vi "Fill.vi"(6 "Color":u32(colorbox), 8 "error in (no error)":errorcluster, 9 "point(x,y)":cluster{"x":i16, "y":i16}, 10 "Ref Color":u32(colorbox), 11 "Data in":T1={"Class"={"Ants"=refnum, "Layer"=refnum, "Templates"=refnum, "Icon"=refnum, "Glyph"=refnum, "Settings"=refnum, "Tools"=refnum}, "Ref"={"Add Layer"=refnum, "Remove Layer"=refnum, "Line Text"=[], "Body Text Spec"=refnum, "DNL_Font"=refnum, "glyph path str"=refnum, "templates path str"=refnum, "Arrow Up"=refnum, "Arrow Down"=refnum, "IE VI Ref"=refnum, "Glyphs tree"=refnum, "Templates tree"=refnum, "Layer Icon Text"=refnum, "Layer Template"=refnum, "Clipboard"=refnum, "BW icon in"=refnum, "Color icon in"=refnum, "Layer Clust"=refnum, "Body Text"=refnum, "DNL_Framework Templates"=refnum, "Search Templates"=refnum, "TextMarker"=refnum, "Tab Control"=refnum, "Search Glyphs"=refnum, "Line Color"=refnum, "DNL_Glyphs []"=refnum, "Fill Color"=refnum, "Tools"=refnum, "Glyphs tree"=refnum, "Icon"=refnum, "Preview"=refnum, "Ants"=refnum, "Terminals"=refnum, "menu reference"=refnum, "LayerNames"=[], "GlyphLoadAnimation"=refnum, "TemplateLoadAnimation"=refnum, "refreshGlyphs"=refnum, "refreshTemplates"=refnum}, "Support"={"AntsRect"={"left"=0, "top"=0, "right"=0, "bottom"=0}, "Mouse Move Coords"={"Horizontal"=0, "Vertical"=0}, "Mouse Down Coords"={"Horizontal"=0, "Vertical"=0}, "Temp Coord"={"Horizontal"=0, "Vertical"=0}, "Action"=enum."Default", "Edge Color"=4914962, "Fill Color"=16860, "Mouse Down?"=FALSE, "Draft Mode?"=FALSE, "Temp Icon"=bytes[3102], "CTRL Pressed"=FALSE, "Move Selection?"=FALSE, "AntsRect Orig"={"left"=0, "top"=0, "right"=0, "bottom"=0}, "Text"="", "TM Set?"=FALSE, "Mouse inside icon?"=FALSE, "Tool (old value)"=0, "Pencil Move Color"=0, "Swap Colors?"=FALSE, "Shift pressed?"=FALSE}}) -> (0 "error out":errorcluster, 3 "Data out":T1={"Class"={"Ants"=refnum, "Layer"=refnum, "Templates"=refnum, "Icon"=refnum, "Glyph"=refnum, "Settings"=refnum, "Tools"=refnum}, "Ref"={"Add Layer"=refnum, "Remove Layer"=refnum, "Line Text"=[], "Body Text Spec"=refnum, "DNL_Font"=refnum, "glyph path str"=refnum, "templates path str"=refnum, "Arrow Up"=refnum, "Arrow Down"=refnum, "IE VI Ref"=refnum, "Glyphs tree"=refnum, "Templates tree"=refnum, "Layer Icon Text"=refnum, "Layer Template"=refnum, "Clipboard"=refnum, "BW icon in"=refnum, "Color icon in"=refnum, "Layer Clust"=refnum, "Body Text"=refnum, "DNL_Framework Templates"=refnum, "Search Templates"=refnum, "TextMarker"=refnum, "Tab Control"=refnum, "Search Glyphs"=refnum, "Line Color"=refnum, "DNL_Glyphs []"=refnum, "Fill Color"=refnum, "Tools"=refnum, "Glyphs tree"=refnum, "Icon"=refnum, "Preview"=refnum, "Ants"=refnum, "Terminals"=refnum, "menu reference"=refnum, "LayerNames"=[], "GlyphLoadAnimation"=refnum, "TemplateLoadAnimation"=refnum, "refreshGlyphs"=refnum, "refreshTemplates"=refnum}, "Support"={"AntsRect"={"left"=0, "top"=0, "right"=0, "bottom"=0}, "Mouse Move Coords"={"Horizontal"=0, "Vertical"=0}, "Mouse Down Coords"={"Horizontal"=0, "Vertical"=0}, "Temp Coord"={"Horizontal"=0, "Vertical"=0}, "Action"=enum."Default", "Edge Color"=4914962, "Fill Color"=16860, "Mouse Down?"=FALSE, "Draft Mode?"=FALSE, "Temp Icon"=bytes[3102], "CTRL Pressed"=FALSE, "Move Selection?"=FALSE, "AntsRect Orig"={"left"=0, "top"=0, "right"=0, "bottom"=0}, "Text"="", "TM Set?"=FALSE, "Mouse inside icon?"=FALSE, "Tool (old value)"=0, "Pencil Move Color"=0, "Swap Colors?"=FALSE, "Shift pressed?"=FALSE}})   [LabVIEW 2021, in "Tools Paint.lvclass"]
uses:
  <resource>/plugins/NIIconEditor/Class/Tools/Tools Paint.lvclass
  <resource>/plugins/NIIconEditor/Controls/IE Data.ctl
  <resource>/plugins/NIIconEditor/Class/Ants/Ants.lvclass
  <resource>/plugins/NIIconEditor/Class/FakedArray/FakedArray.lvclass
  <vilib>/LabVIEW Icon API/lv_icon/Classes/Icon/Icon.lvclass
  <resource>/plugins/NIIconEditor/Class/Icon Library/Glyph.lvclass
  <resource>/plugins/NIIconEditor/Class/Settings/Settings.lvclass
  <resource>/plugins/NIIconEditor/Controls/IE Classes.ctl
  <resource>/plugins/NIIconEditor/Controls/References Cluster.ctl
  <resource>/plugins/NIIconEditor/Controls/SupportClass.ctl
  <vilib>/Utility/miscctls.llb/LVPoint32TypeDef.ctl
  <resource>/plugins/NIIconEditor/Controls/SupportClass_Action.ctl
  <vilib>/LabVIEW Icon API/lv_icon/Controls/IEColor.ctl
  <vilib>/LabVIEW Icon API/lv_icon/Controls/LayerType.ctl
  <vilib>/LabVIEW Icon API/lv_icon/Classes/Layer/Layer.lvclass
  <vilib>/LabVIEW Icon API/lv_icon/Classes/Icon Framework/Icon Framework.lvclass
  C:/projects/labview-icon-editor/source/vi.lib/LabVIEW Icon API/lv_icon/Classes/Layer/Layer.lvclass
  <vilib>/LabVIEW Icon API/lv_icon/lv_icon.lvlib
panel:
  in  "Fill":string="Fill"
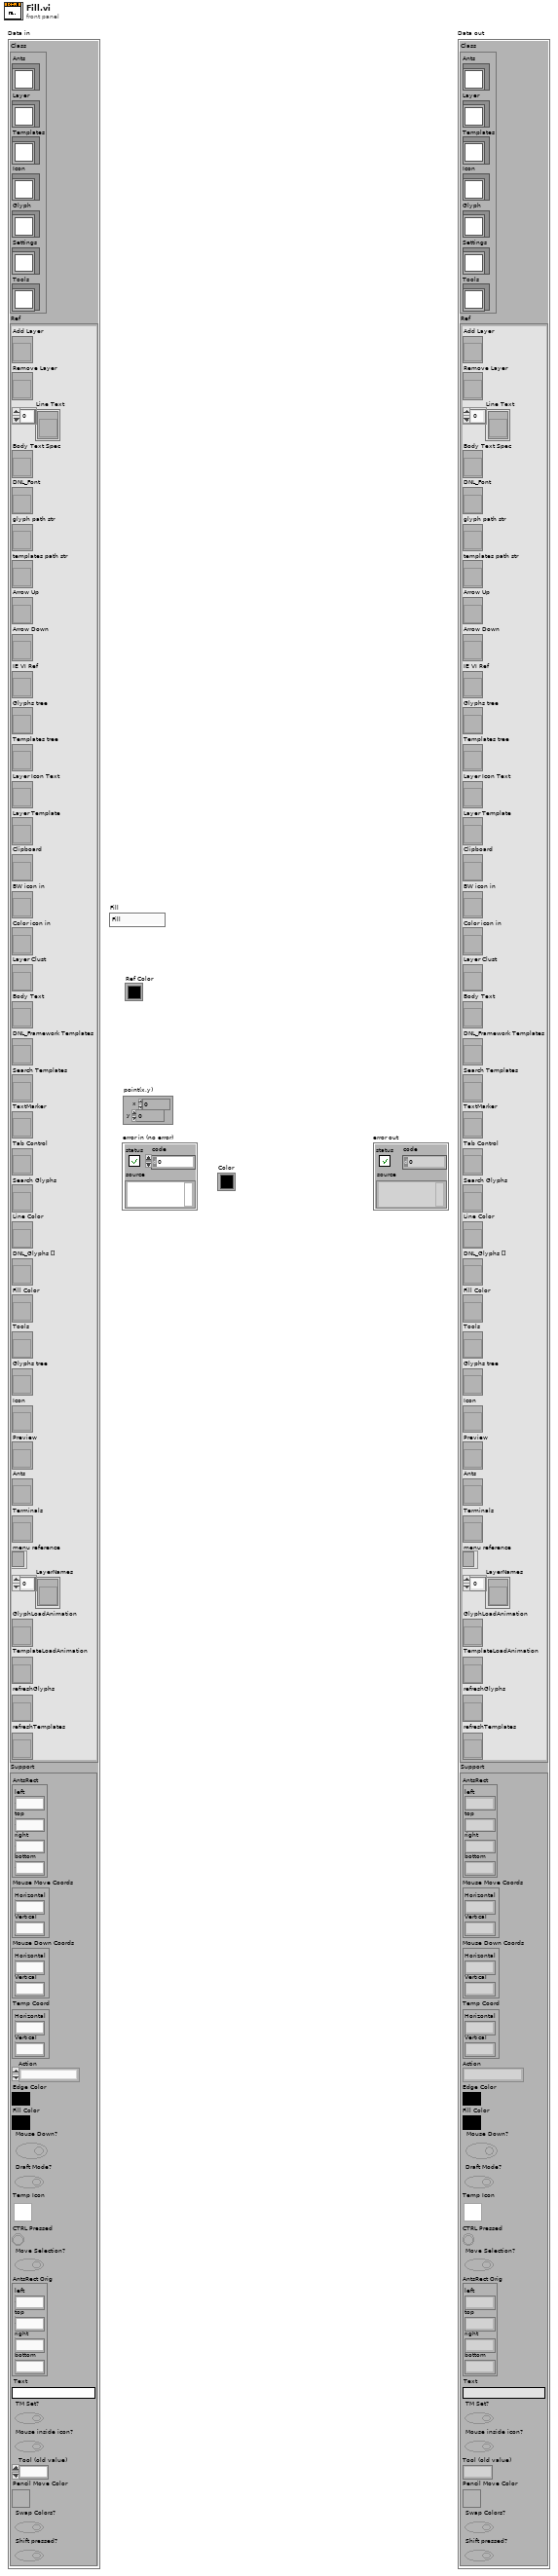
[diagram p1: front panel]
types:
  T1 = typedef "IE Data.ctl" = cluster{"Class":T2, "Ref":T3, "Support":T4}
  T2 = typedef "IE Classes.ctl" = cluster{"Ants":refnum<class "Ants.lvclass">, "Layer":refnum<class "FakedArray.lvclass">, "Templates":refnum<class "FakedArray.lvclass">, "Icon":refnum<class "Icon.lvclass">, "Glyph":refnum<class "Glyph.lvclass">, "Settings":refnum<class "Settings.lvclass">, "Tools":refnum<class "Tools Paint.lvclass">}
  T3 = typedef "References Cluster.ctl" = cluster{"Add Layer":refnum<vi>, "Remove Layer":refnum<vi>, "Line Text":refnum<vi>[], "Body Text Spec":refnum<vi>, "DNL_Font":refnum<vi>, "glyph path str":refnum<vi>, "templates path str":refnum<vi>, "Arrow Up":refnum<vi>, "Arrow Down":refnum<vi>, "IE VI Ref":refnum<vi>, "Glyphs tree":refnum<vi>, "Templates tree":refnum<vi>, "Layer Icon Text":refnum<vi>, "Layer Template":refnum<vi>, "Clipboard":refnum<vi>, "BW icon in":refnum<vi>, "Color icon in":refnum<vi>, "Layer Clust":refnum<vi>, "Body Text":refnum<vi>, "DNL_Framework Templates":refnum<vi>, "Search Templates":refnum<vi>, "TextMarker":refnum<vi>, "Tab Control":refnum<vi>, "Search Glyphs":refnum<vi>, "Line Color":refnum<vi>, "DNL_Glyphs []":refnum<vi>, "Fill Color":refnum<vi>, "Tools":refnum<vi>, "Glyphs tree":refnum<vi>, "Icon":refnum<vi>, "Preview":refnum<vi>, "Ants":refnum<vi>, "Terminals":refnum<vi>, "menu reference":refnum<k9>, "LayerNames":refnum<vi>[], "GlyphLoadAnimation":refnum<vi>, "TemplateLoadAnimation":refnum<vi>, "refreshGlyphs":refnum<vi>, "refreshTemplates":refnum<vi>}
  T4 = typedef "SupportClass.ctl" = cluster{"AntsRect":cluster{"left":i16, "top":i16, "right":i16, "bottom":i16}, "Mouse Move Coords":T5, "Mouse Down Coords":T5, "Temp Coord":T5, "Action":T6, "Edge Color":T7, "Fill Color":T7, "Mouse Down?":bool, "Draft Mode?":bool, "Temp Icon":picture, "CTRL Pressed":bool, "Move Selection?":bool, "AntsRect Orig":cluster{"left":i16, "top":i16, "right":i16, "bottom":i16}, "Text":string, "TM Set?":bool, "Mouse inside icon?":bool, "Tool (old value)":u32, "Pencil Move Color":u32, "Swap Colors?":bool, "Shift pressed?":bool}
  T5 = typedef "LVPoint32TypeDef.ctl" = cluster{"Horizontal":i32, "Vertical":i32}
  T6 = typedef "SupportClass_Action.ctl" = enum16{"Default", "Move Selection", "Glyph Library", "Tool"}
  T7 = typedef "IEColor.ctl" = u32
  T8 = typedef "LayerType.ctl" = enum16{"Graphic", "Text", "Tool", "Graphic Drop"}
  T9 = typedef "INI.ctl" = cluster{"Show Layer Tab?":bool, "Show Terminals?":bool, "Text":cluster{"Font":T10, "Alignment":T11, "Size":T12}, "3rd party Templates":cluster{"Store 3rd party Templates?":bool, "Folder Name":string}, "Merge user layers on commit":bool, "Body Text":T13, "Fill Color":T7, "Edge Color":T7, "Tab":u16, "Tool":T14, "Disable Layers?":bool}
  T10 = typedef "Font.ctl" = string
  T11 = typedef "Alignment.ctl" = u16
  T12 = typedef "Font Size.ctl" = u8
  T13 = typedef "BodyText.ctl" = cluster{"Line 1 text":string, "Line 2 text":string, "Line 3 text":string, "Line 4 text":string, "Line 1 color":u32, "Line 2 color":u32, "Line 3 color":u32, "Line 4 color":u32, "Body Text Spec":cluster{"Font":T10, "Alignment":T11, "Size":u8}, "Center text vertically":bool, "Capitalize Text":bool}
  T14 = typedef "Tools.ctl" = enum32{"Pencil", "Line", "Dropper", "Fill", "Rectangle", "Filled Rectangle", "Ellipse", "Filled Ellipse", "Eraser", "Text", "Select", "Move"}
  T15 = typedef "Layer.ctl" = cluster{"LayerIcon":picture, "LayerName":string, "Opacity":u8, "Visibility?":bool}
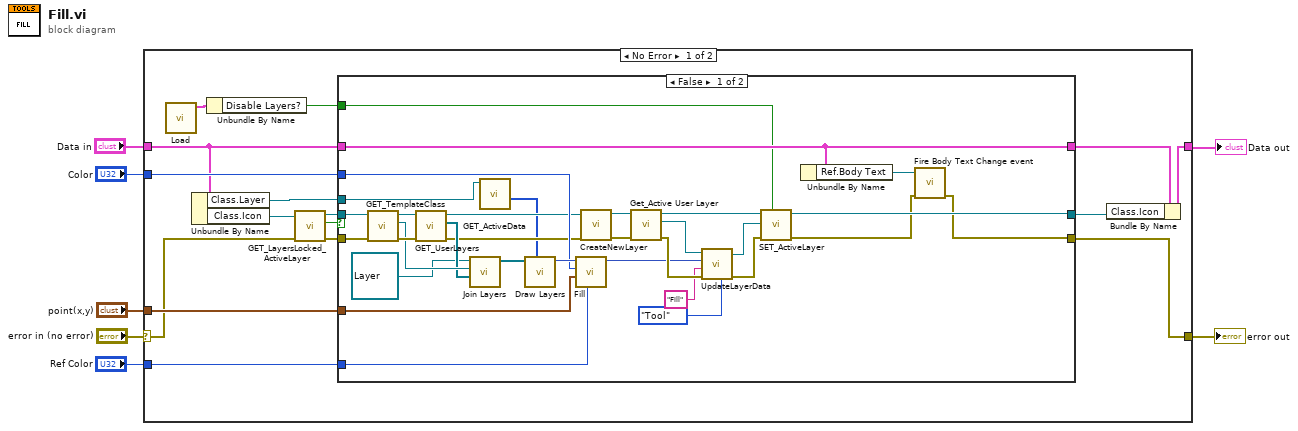
[diagram p0: block diagram]
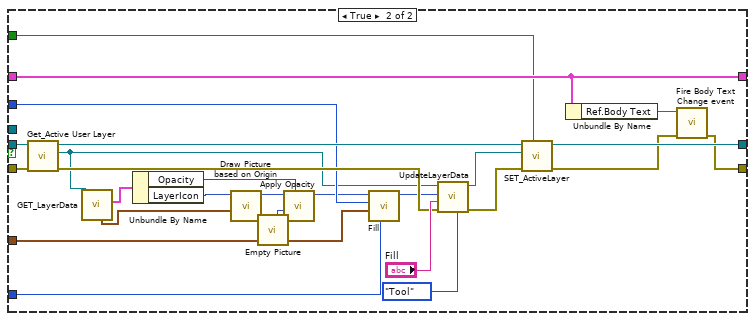
[diagram p2: hidden frame]
diagram:
  n1 = case shown="No Error" "error in (no error)" {
    selector: "error in (no error)" -> [w17 w83]
    tunnel: [w13 w83] -> w6
    tunnel: "point(x,y)" -> [w23 _]
    tunnel: "Color" -> [w19 _]
    tunnel: "Ref Color" -> [w18 _]
    tunnel: "Data in" -> [w15 w82]
    tunnel: [w12 w82] -> w1
    frame No Error {
      n2 = call <resource>:"Load.vi"() -> ("INI Data"=w9:T9)  [unwired: 2 in, 9 out]
      n3 = Unbundle By Name(w15) -> ("Class.Layer"=w10:refnum<class "FakedArray.lvclass">, "Class.Icon"=w16:refnum<class "Icon.lvclass">)
      n4 = Unbundle By Name(w9) -> ("Disable Layers?"=w8:bool)
      n5 = call-dynamic "GET_LayersLocked_ActiveLayer.vi"("error in (no error)"=w17, "Icon.lvclass in"=w16) -> ("error out"=w21:errorcluster, "Layers Locked?"=w20:bool, "Icon.lvclass out"=w22:refnum<class "Icon.lvclass">)  [unwired: 7 out]
      n6 = case shown="False" w20 {
        tunnel: w23 -> [w46 w72]
        tunnel: [w32 w79] -> w11
        tunnel: w22 -> [w54 w81]
        tunnel: w21 -> [w55 w80]
        tunnel: w19 -> [w47 w73]
        tunnel: w18 -> [w48 w71]
        tunnel: [w29 w58] -> w13
        tunnel: w15 -> [w28 w60]
        tunnel: [w28 w60] -> w14
        tunnel: w10 -> [w25 _]
        tunnel: w8 -> [w26 w56]
        frame False {
          n7 = call-dynamic "GET_TemplateClass.vi"("error in (no error)"=w55, "Icon.lvclass in"=w54) -> ("error out"=w53:errorcluster, "Icon Framework.lvclass"=w51:refnum<class "Icon Framework.lvclass">, "Icon.lvclass out"=w52:refnum<class "Icon.lvclass">)  [unwired: 7 out]
          n8 = call-dynamic "GET_UserLayers.vi"("error in (no error)"=w53, "Icon.lvclass in"=w52) -> ("error out"=w34:errorcluster, "All Layers"=w45:refnum<class "Layer.lvclass">[], "Icon.lvclass out"=w35:refnum<class "Icon.lvclass">)  [unwired: 7 out]
          n9 = call <vilib>:"Join Layers.vi"("User Layers"=w45, "Template"=w51, "Icon Text"=refnum<class "Layer.lvclass"> refnum) -> ("Layer out"=w50:refnum<class "Layer.lvclass">[])  [unwired: 3 in, 5 out]
          n10 = call-dynamic "GET_ActiveData.vi"("FakedArray in"=w25) -> ("Active Data []"=w24:i32[])  [unwired: 5 in, 5 out]
          n11 = call <vilib>:"Draw Layers.vi"("Active User Layer Data []"=w24, "Layers"=w50) -> ("Picture"=w49:picture)  [unwired: 3 in, 6 out]
          n12 = call <vilib>:"Fill.vi"("Ref Color"=w48, "Pic Mouse Down"=w46, "New Color"=w47, "Pic In"=w49) -> ("Pic Out"=w33:picture)  [unwired: 3 in, 4 out]
          n13 = call <vilib>:"CreateNewLayer.vi"("error in"=w34, "Icon.lvclass"=w35) -> ("error out"=w43:errorcluster, "Icon.lvclass out"=w44:refnum<class "Icon.lvclass">)  [unwired: 3 in, 5 out]
          n14 = call-dynamic "Get_Active User Layer.vi"("error in (no error)"=w43, "Icon in"=w44) -> ("error out"=w38:errorcluster, "Layer.lvclass"=w42:refnum<class "Layer.lvclass">, "Icon out"=w41:refnum<class "Icon.lvclass">)  [unwired: 7 out]
          n15 = call <vilib>:"UpdateLayerData.vi"("Type"=LayerType."Tool", "error in"=w38, "LayerName"="Fill" ("FileName"), "new picture"=w33, "Active Layer"=w42) -> ("error out"=w39:errorcluster, "Layer.lvclass out"=w40:refnum<class "Layer.lvclass">)  [unwired: 3 in, 2 out]
          n16 = call-dynamic "SET_ActiveLayer.vi"("Combine User Layers?"=w26, "error in (no error)"=w39, "Layer.lvclass"=w40, "Icon.lvclass in"=w41) -> ("error out"=w30:errorcluster, "Icon.lvclass out"=w32:refnum<class "Icon.lvclass">)  [unwired: 6 out]
          n17 = Unbundle By Name(w28) -> ("Ref.Body Text"=w27:refnum<vi>)
          n18 = call <resource>:"Fire Body Text Change event.vi"("error in"=w30, "Ref.Body Text"=w27) -> ("error out"=w29:errorcluster)  [unwired: 2 in, 7 out]
        }
        frame True {
          n19 = call-dynamic "Get_Active User Layer.vi"("error in (no error)"=w80, "Icon in"=w81) -> ("error out"=w75:errorcluster, "Layer.lvclass"=w66:refnum<class "Layer.lvclass">, "Icon out"=w78:refnum<class "Icon.lvclass">)  [unwired: 7 out]
          n20 = call-dynamic "GET_LayerData.vi"("Layer.lvclass in"=w66) -> ("Data"=w65:T15, "Origin"=w63:T5)  [unwired: 1 in, 8 out]
          n21 = Unbundle By Name(w65) -> ("Opacity"=w62:u8, "LayerIcon"=w64:picture)
          n22 = call <vilib>:"Draw Picture based on Origin.vi"("Origin"=w63, "LayerIcon in"=w64) -> ("LayerIcon out"=w67:picture)  [unwired: 1 in, 8 out]
          n23 = call "Empty Picture"() -> ("empty picture"=w68:picture)
          n24 = call <vilib>:"Apply Opacity.vi"("% (100)"=w62, "Bottom"=w68, "Top"=w67) -> ("new picture"=w61:picture)  [unwired: 8 out]
          n25 = call <vilib>:"Fill.vi"("Ref Color"=w71, "Pic Mouse Down"=w72, "New Color"=w73, "Pic In"=w61) -> ("Pic Out"=w70:picture)  [unwired: 3 in, 4 out]
          n26 = call <vilib>:"UpdateLayerData.vi"("Type"=LayerType."Tool", "error in"=w75, "LayerName"="Fill", "new picture"=w70, "Active Layer"=w66) -> ("error out"=w74:errorcluster, "Layer.lvclass out"=w69:refnum<class "Layer.lvclass">)  [unwired: 3 in, 2 out]
          n27 = call-dynamic "SET_ActiveLayer.vi"("Combine User Layers?"=w56, "error in (no error)"=w74, "Layer.lvclass"=w69, "Icon.lvclass in"=w78) -> ("error out"=w59:errorcluster, "Icon.lvclass out"=w79:refnum<class "Icon.lvclass">)  [unwired: 6 out]
          n28 = Unbundle By Name(w60) -> ("Ref.Body Text"=w57:refnum<vi>)
          n29 = call <resource>:"Fire Body Text Change event.vi"("error in"=w59, "Ref.Body Text"=w57) -> ("error out"=w58:errorcluster)  [unwired: 2 in, 7 out]
        }
      }
      n30 = Bundle By Name(cluster=w14, "Class.Icon"=w11) -> (w12:T1)
    }
    frame Error {
    }
  }
  "error out" <- w6
  "Data out" <- w1
